vi "write boolean value .vi"() -> ()   [LabVIEW 2016]
panel:
  in  "Boolean":bool
  in  "stop":bool
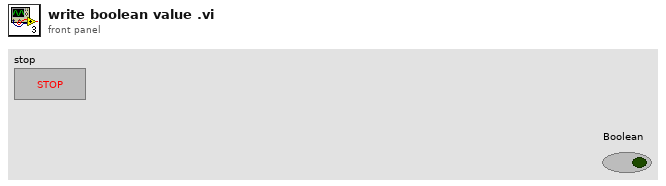
[diagram p1: front panel]
types:
  T1 = enum16{"Read", "Write", "ReadWrite", "BufferedRead", "BufferedReadWrite"}
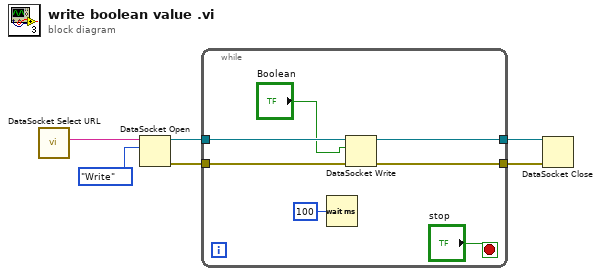
[diagram p0: block diagram]
diagram:
  n1 = call <vilib>:"DataSocket Select URL.vi"() -> ("URL"=w6:string)  [unwired: 9 in, 2 out]
  n2 = DataSocket Open(10:T1."Write" ("mode"), 11:w6) -> (0:w2:errorcluster, 3:w4:refnum<k13>)  [unwired: 2 in]
  n3 = while {
    tunnel: w4 -> [w12]
    tunnel: [w11] -> w3
    tunnel: w2 -> [w10]
    tunnel: [w9] -> w1
    stop <- "stop" stop-if-true
    n4 = Wait (ms)(milliseconds to wait=u32 100) -> ()  [unwired: 1 out]
    n5 = DataSocket Write(8:w10, 10:"Boolean", 11:w12) -> (0:w9:errorcluster, 3:w11:refnum<k13>)  [unwired: 1 in, 1 out]
  }
  n6 = DataSocket Close(8:w1, 11:w3) -> ()  [unwired: 1 in, 2 out]
